vi "parse network message.vi"(8 "error in":errorcluster, 11 "data":string) -> (0 "error out":errorcluster, 3 "message":refnum<class "communicator message.lvclass">)   [LabVIEW 2015, in "TCP server.lvclass"]
uses:
  TCP server.lvclass
  message/communicator message.lvclass
  message/communicator message.lvclass/communicator message.ctl
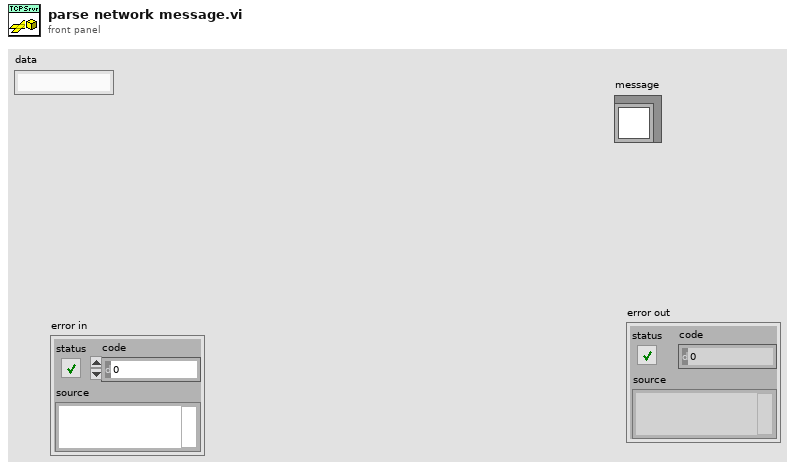
[diagram p1: front panel]
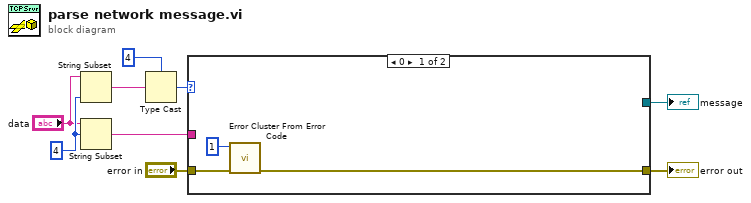
[diagram p0: block diagram]
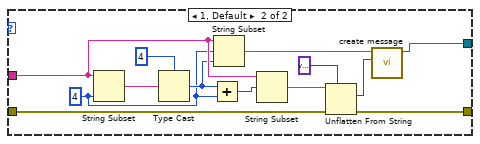
[diagram p2: hidden frame]
diagram:
  w3 = 4 ("length (rest)")
  n1 = String Subset(string="data", length (rest)=w3) -> (substring=w9:string)  [unwired: 1 in]
  n2 = String Subset(string="data", offset (0)=w3) -> (substring=w1:string)  [unwired: 1 in]
  n3 = Type Cast(type=4 ("length (rest)"), x=w9) -> (*(type *) &x=w7:i32)
  n4 = case shown="0" w7 {
    tunnel: [w11 w24] -> w6
    tunnel: "error in" -> [w12 w25]
    tunnel: [_ w13] -> w4
    tunnel: w1 -> [_ w20]
    frame 0 {
      n5 = call <vilib>:"Error Cluster From Error Code.vi"("error in (no error)"=w12, "error code (0)"=1) -> ("error out"=w11:errorcluster)  [unwired: 7 in]
    }
    frame 1, Default {
      w18 = 4 ("offset (0)")
      n6 = String Subset(string=w20, length (rest)=w18) -> (substring=w21:string)  [unwired: 1 in]
      n7 = Type Cast(type=4 ("length (rest)"), x=w21) -> (*(type *) &x=w19:i32)
      n8 = Add(x=w19, y=w18) -> (x+y=w17:i32)
      n9 = String Subset(string=w20, offset (0)=w18, length (rest)=w19) -> (substring=w15:string)
      n10 = String Subset(string=w20, offset (0)=w17) -> (substring=w16:string)  [unwired: 1 in]
      n11 = Unflatten From String(type=variant ("data"), binary string=w16, error in (no error)=w25) -> (value=w14:variant, error out=w24:errorcluster)  [unwired: 2 in, 1 out]
      n12 = call "create message.vi"("data"=w14, "ID"=w15) -> ("message"=w13:refnum<class "communicator message.lvclass">)  [unwired: 9 in]
    }
  }
  "message" <- w4
  "error out" <- w6
